vi "data format.vi"(9 "Q":waveform(dbl), 10 "P":waveform(dbl)) -> (2 "spreadsheet string":string)   [LabVIEW 2014, in "PLS Logging.lvlib"]
uses:
  PLS Logging.lvlib
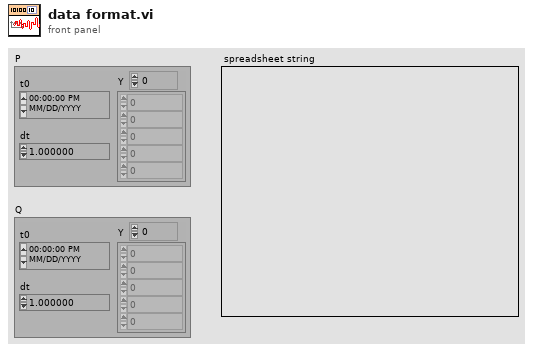
[diagram p1: front panel]
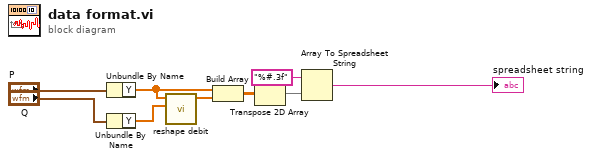
[diagram p0: block diagram]
diagram:
  n1 = Unbundle By Name("P") -> ("Y"=w8:dbl[])
  n2 = Unbundle By Name("Q") -> ("Y"=w7:dbl[])
  n3 = call "reshape debit.vi"("Q"=w7, "P"=w8) -> ("Array"=w9:dbl[])  [unwired: 9 in]
  n4 = Build Array(w8, w9) -> (w3:dbl[][])
  n5 = Transpose 2D Array(2D array=w3) -> (transposed array=w6:dbl[][])
  n6 = Array To Spreadsheet String(array=w6, 3:"%#.3f" ("format string")) -> (spreadsheet string=→"spreadsheet string":string)  [unwired: 1 in]
